vi "Ctor.vi"(8 "error in (no error)":errorcluster, 11 "Terminal in":refnum<class "Terminal.lvclass">) -> (0 "error out":errorcluster, 3 "Terminal out":refnum<class "Terminal.lvclass">)   [LabVIEW 2020, in "PicoG-Processor.lvlib" / "Terminal.lvclass"]
uses:
  Terminal.lvclass
  <vilib>/IlluminatedG/IG OOPanel/OOPanel/Panel/Panel.lvclass
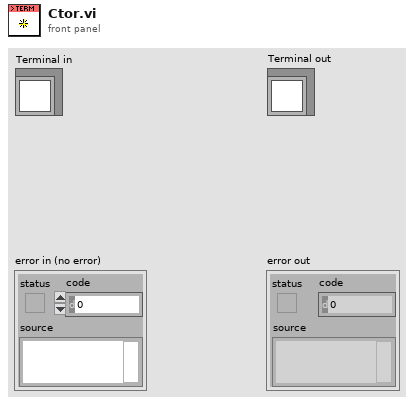
[diagram p1: front panel]
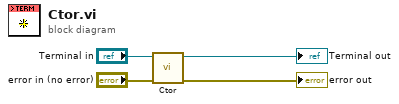
[diagram p0: block diagram]
diagram:
  n1 = call-parent "Ctor.vi"("error in (no error)"="error in (no error)", "Panel in"="Terminal in") -> ("error out"=→"error out":errorcluster, "Panel out"=→"Terminal out":refnum<class "Terminal.lvclass">)  [unwired: 8 in]
